vi "axis_GetHttpRequest.vi"(6 "Frame Rate":u32(slide) max=30 scale=0.0..30.0, 7 "Compression":u32(slide)=25 scale=0.0..99.0, 10 "Color?":bool=TRUE, 11 "Pixel Format":T1(ring)) -> (3 "HTTP Request":string)   [LabVIEW 2009]
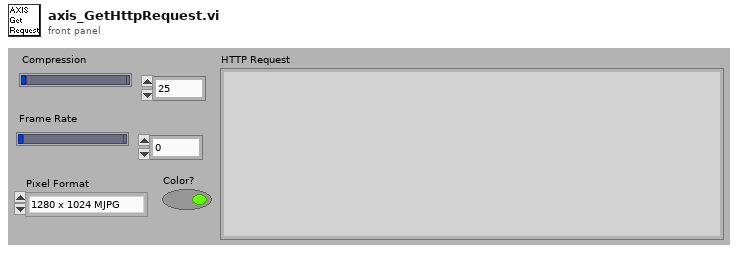
[diagram p1: front panel]
types:
  T1 = enum16{"1280 x 1024 MJPG", "1280 x 960 MJPG", "1280 x 720 MJPG", "1280 x 480 MJPG", "640 x 480 MJPG", "320 x 240 MJPG", "160 x 120 MJPG"}
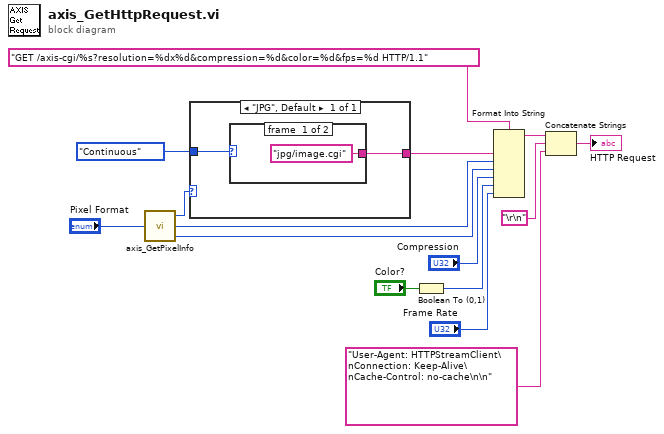
[diagram p0: block diagram]
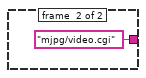
[diagram p2: hidden frame]
diagram:
  n1 = call "axis_GetPixelInfo.vi"("Pixel Format"="Pixel Format") -> ("Type"=w7:enum16{"JPG"}, "Width"=w14:u32, "Height"=w15:u32)
  n2 = case shown="\"JPG\", Default" w7 {
    tunnel: [w17] -> w3
    tunnel: enum16{"SingleShot", "Continuous"}."Continuous" ("Acquisition Type") -> [w16]
    frame "JPG", Default {
      n3 = case shown="\"Continuous\"" w16 {
        tunnel: ["jpg/image.cgi" "mjpg/video.cgi"] -> w17
        frame #0 {
        }
        frame #1 {
        }
      }
    }
  }
  n4 = Boolean To (0,1)(Boolean="Color?") -> (0, 1=w4:i16)
  n5 = Format Into String(format string="GET /axis-cgi/%s?resolution=%dx%d&compression=%d&color=%d&fps=%d HTTP/1.1", w3, w14, w15, "Compression", w4, "Frame Rate") -> (resulting string=w9:string)  [unwired: 2 in, 1 out]
  n6 = Concatenate Strings(w9, "\r\n", "User-Agent: HTTPStreamClient\nConnection: Keep-Alive\nCache-Control: no-cache\n\n") -> (→"HTTP Request":string)
